vi "Get Actor Data.vi"(8 "error in (no error)":errorcluster, 10 "Actor's Self Q":refnum<class "Message Enqueuer.lvclass">, 11 "Monitor Data in":refnum<class "Monitor Data.lvclass">) -> (0 "error out":errorcluster, 1 "Nested Actors":refnum<class "Message Enqueuer.lvclass">[](array[class]), 2 "Actor Data":T1={"Actor Type"="", "Actor Core VI"="", "Self"=refnum, "Caller"=refnum, "Actor Label"="", "Last Ping"=-1.0}, 3 "Monitor Data out":refnum<class "Monitor Data.lvclass">, 4 "Found?":bool)   [LabVIEW 2020, in "Monitor Data.lvclass"]
doc: "Returns information about the specified actor\n\nCopyright: MGI 2016\nAuthor: Derek Trepanier"
uses:
  <vilib>/MGI/Monitored Actor/Monitor Data/Monitor Data.lvclass
  <vilib>/ActorFramework/Message Enqueuer/Message Enqueuer.lvclass
  <vilib>/MGI/Monitored Actor/Monitor Data/Actor Data.ctl
  <vilib>/MGI/Monitored Actor/Monitor Data/Monitor Data.lvclass/Monitor Data.ctl
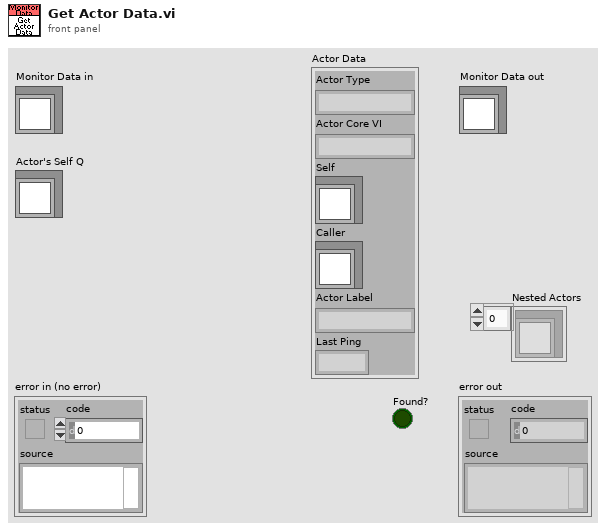
[diagram p1: front panel]
types:
  T1 = typedef "Monitor Data.lvclass/Actor Data.ctl" = cluster{"Actor Type":string, "Actor Core VI":string, "Self":refnum<class "Message Enqueuer.lvclass">, "Caller":refnum<class "Message Enqueuer.lvclass">, "Actor Label":string, "Last Ping":dbl}
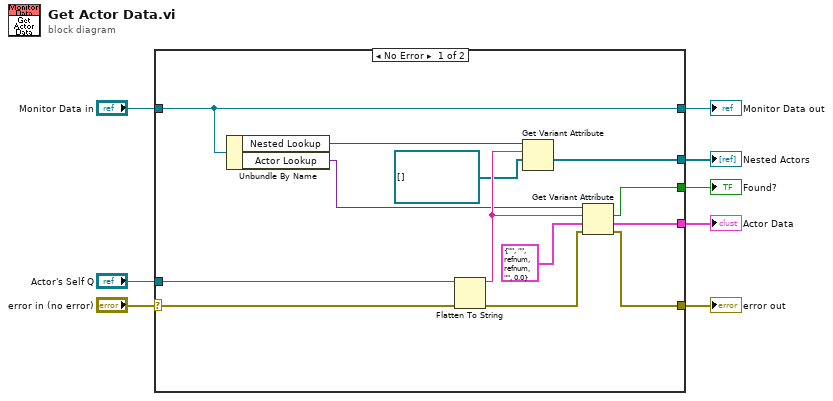
[diagram p0: block diagram]
diagram:
  n1 = case shown="No Error" "error in (no error)" {
    selector: "error in (no error)" -> [w11 w23]
    tunnel: [w12 w23] -> w7
    tunnel: [w20 w22] -> w5
    tunnel: "Monitor Data in" -> [w20 w22]
    tunnel: "Actor's Self Q" -> [w21 _]
    tunnel: [w19 _] -> w3
    tunnel: [w10 _] -> w2
    tunnel: [w9 _] -> w1
    frame No Error {
      n2 = Unbundle By Name(w20) -> ("Nested Lookup"=w14:variant, "Actor Lookup"=w13:variant)
      n3 = Flatten To String(anything=w21, error in (no error)=w11) -> (data string=w16:string, error out=w17:errorcluster)  [unwired: 2 in, 1 out]
      n4 = Get Variant Attribute(Variant=w14, name=w16, default value (empty Variant)=refnum<class "Message Enqueuer.lvclass">[] []) -> (value=w19:refnum<class "Message Enqueuer.lvclass">[])  [unwired: 1 in, 3 out]
      n5 = Get Variant Attribute(Variant=w13, name=w16, default value (empty Variant)=T1 {"Actor Type"="", "Actor Core VI"="", "Self"=refnum, "Caller"=refnum, "Actor Label"="", "Last Ping"=0.0} ("Actor Data"), error in=w17) -> (found=w9:bool, value=w10:T1, error out=w12:errorcluster)  [unwired: 1 out]
    }
    frame Error {
    }
  }
  "error out" <- w7
  "Monitor Data out" <- w5
  "Nested Actors" <- w3
  "Actor Data" <- w2
  "Found?" <- w1
